vi "ilamparidi sankar.vi"() -> ()   [LabVIEW 2018]
uses:
  <vilib>/sound2/lvsound2.llb/Sound Data Format.ctl
  <vilib>/sound2/lvsound2.llb/Sound Input Read (DBL).vi
  <vilib>/sound2/lvsound2.llb/Sound Output Write (DBL).vi
  <vilib>/sound2/lvsound2.llb/Sound Output Set Volume (Single).vi
  <vilib>/measure/matone.llb/Extract Single Tone Information N Chan.vi
  <vilib>/measure/NI_MAPro.lvlib
panel:
  out "Boolean 3":bool
  out "Boolean 2":bool
  out "Boolean":bool
  in  "Lower Cut-Off":dbl(slide)=8.0 scale=0.0..100.0
  out "Filtered Signal":dynamicdata(graph)
  out "detected":dbl[](graph)
  out "detected amplitudes":dbl[](array[numeric]) format="%.2p"
  out "detected frequencies":dbl[](array[numeric]) format="%.2p"
  out "actually frequency":waveform(dbl)[](graph)
  in  "sound format":T1={"sample rate (S/s)"=22050.0, "number of channels"=2, "bits per sample"=16}
  in  "volume":dbl(slide)=100.0 scale=0.0..100.0
  in  "stop":bool
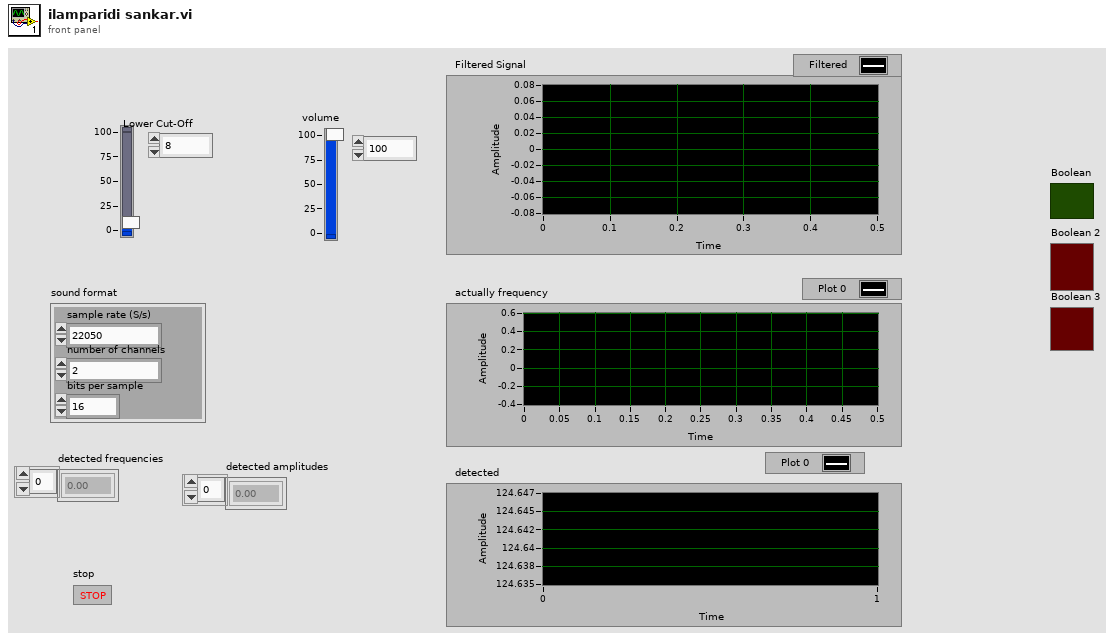
[diagram p1: front panel]
types:
  T1 = typedef "Sound Data Format.ctl" = cluster{"sample rate (S/s)":dbl, "number of channels":i32, "bits per sample":i32}
  T2 = typedef "Sound Input Task ID.ctl" = u32
  T3 = typedef "Sound Output Task ID.ctl" = u32
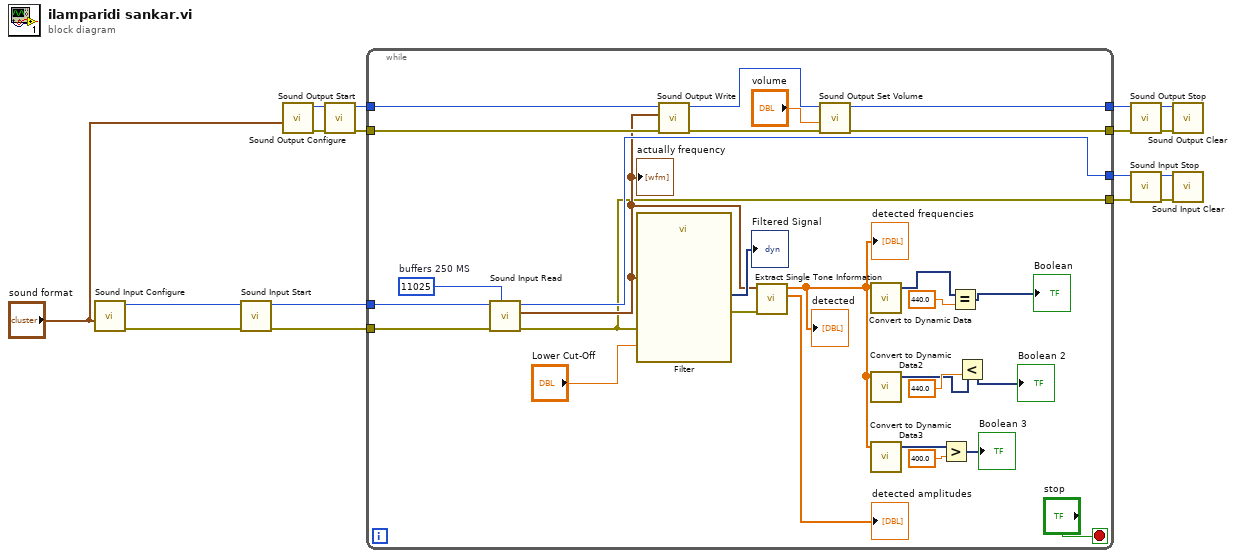
[diagram p0: block diagram]
diagram:
  n1 = call <vilib>:"Sound Input Configure.vi"("sound format"="sound format") -> ("error out"=w16:errorcluster, "task ID"=w17:T2)  [unwired: 9 in]
  n2 = call <vilib>:"Sound Input Start.vi"("error in (no error)"=w16, "task ID"=w17) -> ("error out"=w14:errorcluster, "task ID out"=w15:T2)  [unwired: 8 in]
  n3 = call <vilib>:"Sound Output Configure.vi"("sound format"="sound format") -> ("error out"=w13:errorcluster, "task ID"=w12:T3)  [unwired: 9 in]
  n4 = call <vilib>:"Sound Output Start.vi"("error in (no error)"=w13, "task ID"=w12) -> ("error out"=w10:errorcluster, "task ID out"=w11:T3)  [unwired: 8 in]
  n5 = while {
    tunnel: w15 -> [w45]
    tunnel: w14 -> [w44]
    tunnel: [w42] -> w9
    tunnel: [w28] -> w8
    tunnel: w11 -> [w34]
    tunnel: w10 -> [w35]
    tunnel: [w37] -> w5
    tunnel: [w36] -> w4
    stop <- "stop" stop-if-true
    w43 = 11025  # buffers 250 MS
    n6 = call-poly <vilib>:"Sound Input Read.vi"("number of samples/ch"=w43, "error in (no error)"=w44, "task ID"=w45) -> ("error out"=w28:errorcluster, "data"=w30:waveform(dbl)[], "task ID out"=w42:T2)  [unwired: 6 in]
    "actually frequency" <- w30
    n7 = call "Filter"("error in (no error)"=w28, "Lower Cut-Off"="Lower Cut-Off", "Signal"=w30) -> ("error out"=w29:errorcluster, "Filtered Signal"=→"Filtered Signal":dynamicdata)  [unwired: 7 in]
    n8 = call-poly <vilib>:"Sound Output Write.vi"("error in (no error)"=w35, "data"=w30, "task ID"=w34) -> ("error out"=w39:errorcluster, "task ID out"=w40:T3)  [unwired: 7 in]
    n9 = call-poly <vilib>:"Extract Single Tone Information.vi"("error in (no error)"=w29, "time signals in"=w30) -> ("detected amplitudes"=→"detected amplitudes":dbl[], "detected frequencies"=w25:dbl[])  [unwired: 4 in, 4 out]
    "detected frequencies" <- w25
    "detected" <- w25
    n10 = call-poly <vilib>:"Sound Output Set Volume.vi"("error in (no error)"=w39, "volume"="volume", "task ID"=w40) -> ("error out"=w37:errorcluster, "task ID out"=w36:T3)  [unwired: 7 in]
    n11 = call "Convert to Dynamic Data"("Array"=w25) -> ("Dynamic Data Type"=w19:dynamicdata)  [unwired: 3 in]
    n12 = call "Convert to Dynamic Data2"("Array"=w25) -> ("Dynamic Data Type"=w22:dynamicdata)  [unwired: 3 in]
    n13 = call "Convert to Dynamic Data3"("Array"=w25) -> ("Dynamic Data Type"=w27:dynamicdata)  [unwired: 3 in]
    n14 = Greater?(x=w27, y=400.0) -> (0:→"Boolean 3":dynamicdata)
    n15 = Equal?(x=w19, y=440.0) -> (x = y?=→"Boolean":dynamicdata)
    n16 = Less?(x=w22, y=440.0) -> (x < y?=→"Boolean 2":dynamicdata)
  }
  n17 = call <vilib>:"Sound Output Stop.vi"("error in (no error)"=w5, "task ID"=w4) -> ("error out"=w1:errorcluster, "task ID out"=w2:T3)  [unwired: 8 in]
  n18 = call <vilib>:"Sound Input Stop.vi"("error in (no error)"=w8, "task ID"=w9) -> ("error out"=w6:errorcluster, "task ID out"=w7:T2)  [unwired: 8 in]
  n19 = call <vilib>:"Sound Output Clear.vi"("error in (no error)"=w1, "task ID"=w2) -> ()  [unwired: 9 in, 1 out]
  n20 = call <vilib>:"Sound Input Clear.vi"("error in (no error)"=w6, "task ID"=w7) -> ()  [unwired: 9 in, 1 out]
